vi "Save_Data_To_File.vi"(8 "error in (no error)":errorcluster, 11 "Analysis in":refnum<class "Analysis.lvclass">) -> (0 "error out":errorcluster, 3 "Analysis out":refnum<class "Analysis.lvclass">)   [LabVIEW 2017]
uses:
  Classes/Analysis/Analysis.lvclass
  global variables.vi
  Classes/StatusLog/StatusLog.lvclass
  Classes/DataLoggingText/DataLogging.lvclass
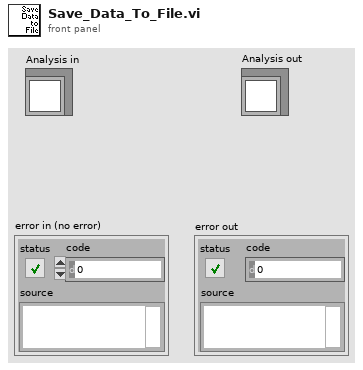
[diagram p1: front panel]
types:
  T1 = typedef "StandardDataArray_new.ctl" = string[][]
  T2 = typedef "PipetteDataArray.ctl" = string[][]
  T3 = typedef "CounterArray.ctl" = string[][]
  T4 = typedef "ScanDataArray_new.ctl" = cluster{"scan data":string[][]}[]
  T5 = typedef "PeakCenterArray.ctl" = string[][]
  T6 = typedef "AnalysisDataArray.ctl" = cluster{"analysis data":string[][]}[]
  T7 = typedef "ExtrapolationResultsArray.ctl" = string[][]
  T8 = typedef "SystemDeviceDataArray.ctl" = cluster{"device data":string[][]}[]
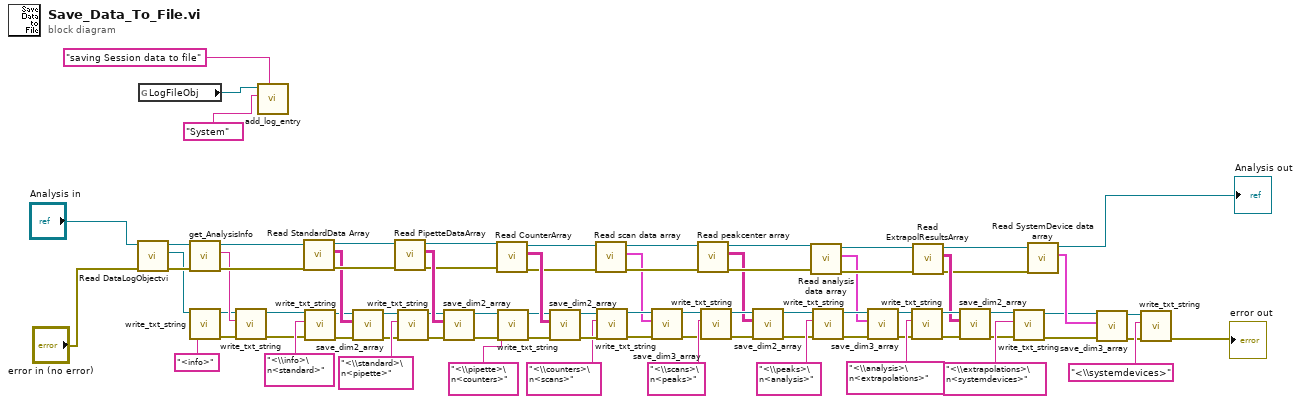
[diagram p0: block diagram]
diagram:
  n1 = call-dynamic "Read DataLogObjectvi.vi"("error in (no error)"="error in (no error)", "Analysis in"="Analysis in") -> ("error out"=w41:errorcluster, "DataLogging.lvclass"=w39:refnum<class "DataLogging.lvclass">, "Analysis out"=w40:refnum<class "Analysis.lvclass">)  [unwired: 7 in]
  n2 = global read "global variables.vi" "LogFileObj"() -> (w13:refnum<class "StatusLog.lvclass">)
  n3 = call "get_AnalysisInfo.vi"("error in (no error)"=w41, "Analysis in"=w40) -> ("error out"=w68:errorcluster, "AnalysisInfo out"=w45:string, "Analysis out"=w67:refnum<class "Analysis.lvclass">)  [unwired: 7 in]
  n4 = call-dynamic "write_txt_string.vi"("data string"="<info>", "DataLoggingText in"=w39) -> ("error out"=w43:errorcluster, "DataLoggingText out"=w42:refnum<class "DataLogging.lvclass">)  [unwired: 8 in]
  n5 = call-dynamic "write_txt_string.vi"("error in (no error)"=w43, "data string"=w45, "DataLoggingText in"=w42) -> ("error out"=w62:errorcluster, "DataLoggingText out"=w61:refnum<class "DataLogging.lvclass">)  [unwired: 7 in]
  n6 = call-dynamic "add_log_entry.vi"("new entry"="saving Session data to file" ("format string"), "log identifiers"="System", "StatusLog in"=w13) -> ()  [unwired: 5 in, 2 out]
  n7 = call-dynamic "Read StandardData Array.vi"("error in (no error)"=w68, "Analysis in"=w67) -> ("error out"=w75:errorcluster, "StandardData Array"=w69:T1, "Analysis out"=w74:refnum<class "Analysis.lvclass">)  [unwired: 7 in]
  n8 = call-dynamic "write_txt_string.vi"("error in (no error)"=w62, "data string"="<\\info>\n<standard>", "DataLoggingText in"=w61) -> ("error out"=w59:errorcluster, "DataLoggingText out"=w60:refnum<class "DataLogging.lvclass">)  [unwired: 7 in]
  n9 = call "save_dim2_array.vi"("error in (no error)"=w59, "2dim data array"=w69, "DataLogging in"=w60) -> ("error out"=w64:errorcluster, "DataLogging out"=w63:refnum<class "DataLogging.lvclass">)  [unwired: 7 in]
  n10 = call-dynamic "Read PipetteDataArray.vi"("error in (no error)"=w75, "Analysis in"=w74) -> ("error out"=w77:errorcluster, "PipetteDataArray"=w78:T2, "Analysis out"=w76:refnum<class "Analysis.lvclass">)  [unwired: 7 in]
  n11 = call-dynamic "write_txt_string.vi"("error in (no error)"=w64, "data string"="<\\standard>\n<pipette>", "DataLoggingText in"=w63) -> ("error out"=w70:errorcluster, "DataLoggingText out"=w71:refnum<class "DataLogging.lvclass">)  [unwired: 7 in]
  n12 = call "save_dim2_array.vi"("error in (no error)"=w70, "2dim data array"=w78, "DataLogging in"=w71) -> ("error out"=w73:errorcluster, "DataLogging out"=w72:refnum<class "DataLogging.lvclass">)  [unwired: 7 in]
  n13 = call-dynamic "Read CounterArray.vi"("error in (no error)"=w77, "Analysis in"=w76) -> ("error out"=w56:errorcluster, "CounterArray"=w57:T3, "Analysis out"=w55:refnum<class "Analysis.lvclass">)  [unwired: 7 in]
  n14 = call-dynamic "write_txt_string.vi"("error in (no error)"=w73, "data string"="<\\pipette>\n<counters>", "DataLoggingText in"=w72) -> ("error out"=w50:errorcluster, "DataLoggingText out"=w51:refnum<class "DataLogging.lvclass">)  [unwired: 7 in]
  n15 = call "save_dim2_array.vi"("error in (no error)"=w50, "2dim data array"=w57, "DataLogging in"=w51) -> ("error out"=w53:errorcluster, "DataLogging out"=w52:refnum<class "DataLogging.lvclass">)  [unwired: 7 in]
  n16 = call-dynamic "Read scan data array.vi"("error in (no error)"=w56, "Analysis in"=w55) -> ("error out"=w17:errorcluster, "scan data array"=w15:T4, "Analysis out"=w16:refnum<class "Analysis.lvclass">)  [unwired: 7 in]
  n17 = call-dynamic "write_txt_string.vi"("error in (no error)"=w53, "data string"="<\\counters>\n<scans>", "DataLoggingText in"=w52) -> ("error out"=w58:errorcluster, "DataLoggingText out"=w25:refnum<class "DataLogging.lvclass">)  [unwired: 7 in]
  n18 = call "save_dim3_array.vi"("error in (no error)"=w58, "ana/scan data array"=w15, "DataLogging in"=w25) -> ("error out"=w27:errorcluster, "DataLogging out"=w26:refnum<class "DataLogging.lvclass">)  [unwired: 7 in]
  n19 = call-dynamic "Read peakcenter array.vi"("error in (no error)"=w17, "Analysis in"=w16) -> ("error out"=w20:errorcluster, "peakcenter array"=w18:T5, "Analysis out"=w19:refnum<class "Analysis.lvclass">)  [unwired: 7 in]
  n20 = call-dynamic "write_txt_string.vi"("error in (no error)"=w27, "data string"="<\\scans>\n<peaks>", "DataLoggingText in"=w26) -> ("error out"=w29:errorcluster, "DataLoggingText out"=w28:refnum<class "DataLogging.lvclass">)  [unwired: 7 in]
  n21 = call "save_dim2_array.vi"("error in (no error)"=w29, "2dim data array"=w18, "DataLogging in"=w28) -> ("error out"=w30:errorcluster, "DataLogging out"=w31:refnum<class "DataLogging.lvclass">)  [unwired: 7 in]
  n22 = call-dynamic "Read analysis data array.vi"("error in (no error)"=w20, "Analysis in"=w19) -> ("error out"=w23:errorcluster, "analysis data array"=w21:T6, "Analysis out"=w22:refnum<class "Analysis.lvclass">)  [unwired: 7 in]
  n23 = call-dynamic "write_txt_string.vi"("error in (no error)"=w30, "data string"="<\\peaks>\n<analysis>", "DataLoggingText in"=w31) -> ("error out"=w33:errorcluster, "DataLoggingText out"=w32:refnum<class "DataLogging.lvclass">)  [unwired: 7 in]
  n24 = call "save_dim3_array.vi"("error in (no error)"=w33, "ana/scan data array"=w21, "DataLogging in"=w32) -> ("error out"=w35:errorcluster, "DataLogging out"=w34:refnum<class "DataLogging.lvclass">)  [unwired: 7 in]
  n25 = call-dynamic "write_txt_string.vi"("error in (no error)"=w35, "data string"="<\\analysis>\n<extrapolations>", "DataLoggingText in"=w34) -> ("error out"=w37:errorcluster, "DataLoggingText out"=w36:refnum<class "DataLogging.lvclass">)  [unwired: 7 in]
  n26 = call-dynamic "Read ExtrapolResultsArray.vi"("error in (no error)"=w23, "Analysis in"=w22) -> ("error out"=w9:errorcluster, "ExtrapolResultsArray"=w24:T7, "Analysis out"=w10:refnum<class "Analysis.lvclass">)  [unwired: 7 in]
  n27 = call "save_dim2_array.vi"("error in (no error)"=w37, "2dim data array"=w24, "DataLogging in"=w36) -> ("error out"=w80:errorcluster, "DataLogging out"=w79:refnum<class "DataLogging.lvclass">)  [unwired: 7 in]
  n28 = call-dynamic "write_txt_string.vi"("error in (no error)"=w80, "data string"="<\\extrapolations>\n<systemdevices>", "DataLoggingText in"=w79) -> ("error out"=w2:errorcluster, "DataLoggingText out"=w3:refnum<class "DataLogging.lvclass">)  [unwired: 7 in]
  n29 = call-dynamic "Read SystemDevice data array.vi"("error in (no error)"=w9, "Analysis in"=w10) -> ("SystemDevice data array"=w4:T8, "Analysis out"=→"Analysis out":refnum<class "Analysis.lvclass">)  [unwired: 7 in, 1 out]
  n30 = call "save_dim3_array.vi"("error in (no error)"=w2, "ana/scan data array"=w4, "DataLogging in"=w3) -> ("error out"=w6:errorcluster, "DataLogging out"=w5:refnum<class "DataLogging.lvclass">)  [unwired: 7 in]
  n31 = call-dynamic "write_txt_string.vi"("error in (no error)"=w6, "data string"="<\\systemdevices>", "DataLoggingText in"=w5) -> ("error out"=→"error out":errorcluster)  [unwired: 7 in, 1 out]
